vi "Add License to All Project VIs.vi"(8 "error in (no error)":errorcluster, 10 "License Text to Add":string, 11 "VI in":refnum<vi>) -> (0 "error out":errorcluster)   [LabVIEW 2020, in "Add License to VI Documentation.lvlib"]
uses:
  Add License to VI Documentation.lvlib
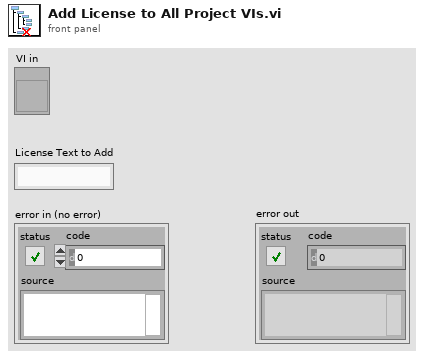
[diagram p1: front panel]
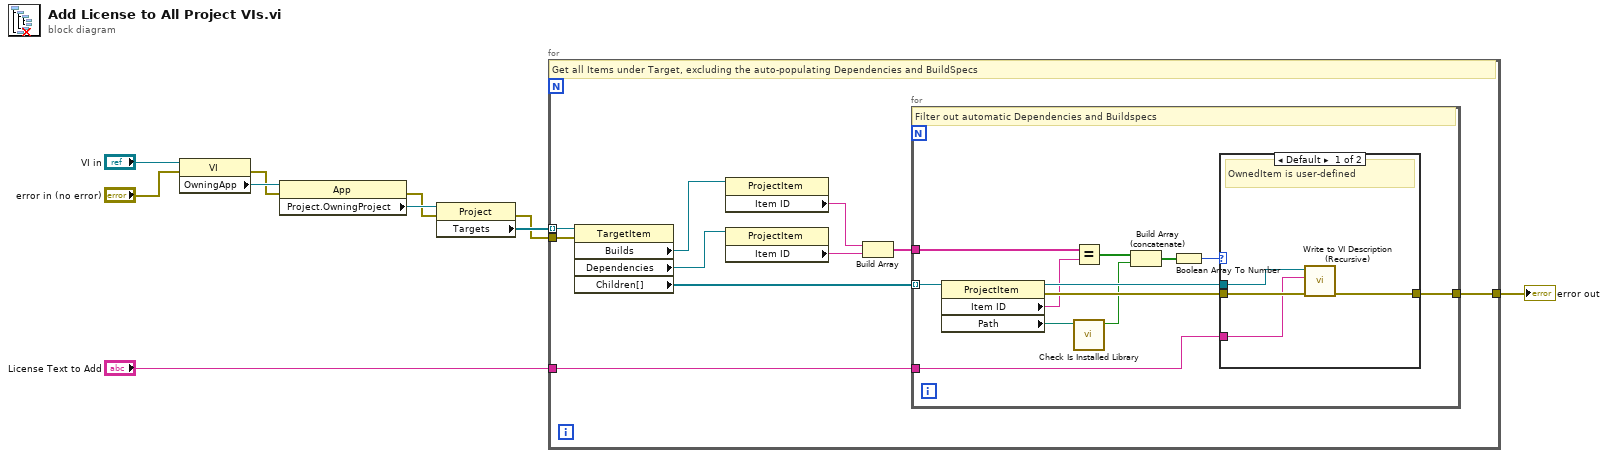
[diagram p0: block diagram]
diagram:
  n1 = property class="VI"(reference="VI in", error in="error in (no error)") -> (error out=w5:errorcluster, "OwningApp"=w8:refnum<vi>)  [unwired: 1 out]
  n2 = property class="App"(reference=w8, error in=w5) -> (error out=w4:errorcluster, "Project.OwningProject"=w7:refnum<vi>)  [unwired: 1 out]
  n3 = property class="Project"(reference=w7, error in=w4) -> (error out=w3:errorcluster, "Targets"=w6:refnum<vi>[])  [unwired: 1 out]
  n4 = for {
    tunnel: w6 -> [w20] mode=indexing
    tunnel: w3 -> [w13]
    tunnel: "License Text to Add" -> [w12]
    tunnel: [w11] -> w1
    # "Get all Items under Target, excluding the auto-populating Dependencies and BuildSpecs"
    n5 = property class="TargetItem"(reference=w20, error in=w13) -> ("Builds"=w17:refnum<vi>, "Dependencies"=w18:refnum<vi>, "Children[]"=w19:refnum<vi>[])  [unwired: 2 out]
    n6 = property class="ProjectItem"(reference=w17) -> ("Item ID"=w15:string)  [unwired: 1 in, 2 out]
    n7 = property class="ProjectItem"(reference=w18) -> ("Item ID"=w16:string)  [unwired: 1 in, 2 out]
    n8 = Build Array(w15, w16) -> (w14:string[])
    n9 = for {
      tunnel: w19 -> [w32] mode=indexing
      tunnel: w14 -> [w30]
      tunnel: w12 -> [w26]
      tunnel: [w25] -> w11
      # "Filter out automatic Dependencies and Buildspecs"
      n10 = property class="ProjectItem"(reference=w32) -> (reference out=w31:refnum<vi>, error out=w27:errorcluster, "Item ID"=w21:string, "Path"=w24:path)  [unwired: 1 in]
      n11 = Equal?(x=w30, y=w21) -> (x = y?=w29:bool[])
      n12 = call "Check Is Installed Library.vi"("Item Path"=w24) -> ("Is Installed Library?"=w22:bool)  [unwired: 9 in, 1 out]
      n13 = Build Array (concatenate)(w29, w22) -> (w23:bool[])
      n14 = Boolean Array To Number(Boolean array=w23) -> (number=w28:u32)
      n15 = case shown="Default" w28 {
        tunnel: w31 -> [w36 _]
        tunnel: w27 -> [w35 w37]
        tunnel: [w34 w37] -> w25
        tunnel: w26 -> [w33 _]
        frame Default {
          # "OwnedItem is user-defined"
          n16 = call "Write to VI Description (Recursive).vi"("error in (no error)"=w35, "License Text to Add"=w33, "ProjectItem in"=w36) -> ("error out"=w34:errorcluster)  [unwired: 8 in]
        }
        frame 1.. {
          # "...or item lives inside\ninstalled libraries folder\n(vi.lib, user.lib, instr.lib)"
          # "In BuildSpecs or Dependencies"
        }
      }
    }
  }
  "error out" <- w1
